vi "Part 2.vi"(11 "Input":string) -> (3 "Output":i64)   [LabVIEW 2021]
uses:
  <userlib>/_OpenG.lib/string/string.llb/Convert EOLs (String)__ogtk.vi
  Module/Module.lvclass
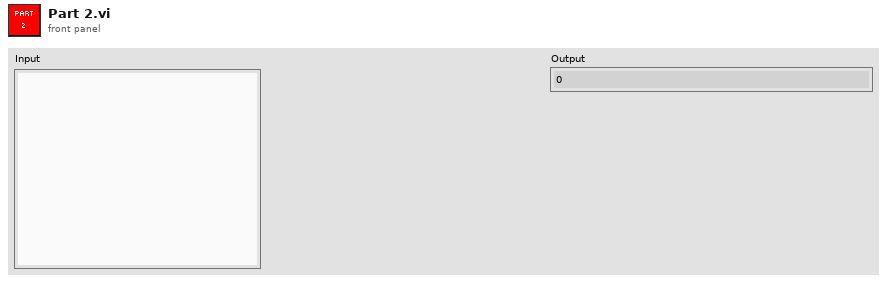
[diagram p1: front panel]
types:
  T1 = cluster{"From":string, "To":string, "Pulse":bool}
  T2 = cluster{"From":string, "To":string, "Pulse":bool}[]
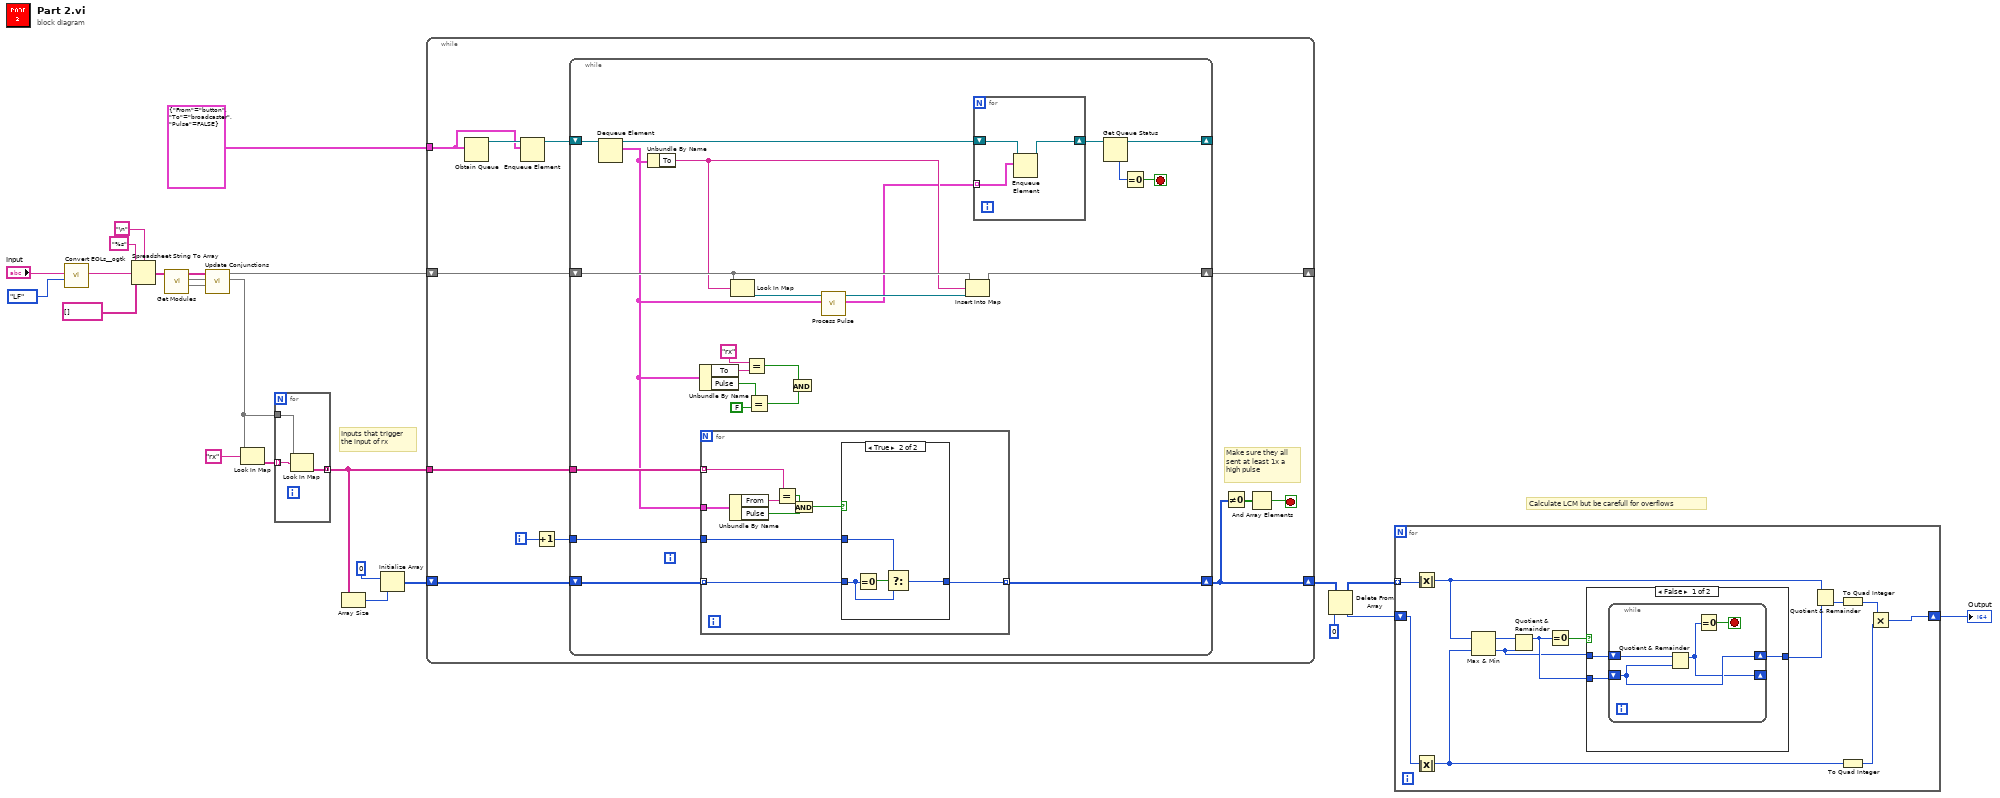
[diagram p0: block diagram]
diagram:
  # "Inputs that trigger\nthe input of rx"
  # "Calculate LCM but be carefull for overflows"
  n1 = call-poly <userlib>:"Convert EOLs__ogtk.vi"("Convert to:"=enum16{"CR", "LF", "CRLF"}."LF", "String in"="Input") -> ("String out"=w20:string)  [unwired: 9 in]
  n2 = Spreadsheet String To Array(delimiter (Tab)="\n", format string="%s", spreadsheet string=w20, array type (2D Dbl)=string[] []) -> (array=w18:string[])
  n3 = call "Get Modules.vi"("Module list in"=w18) -> ("Destination Map"=w15:map{string, string[]}, "Module Map"=w16:map{string, refnum<class "Module.lvclass">}, "Conjunctions out"=w17:string[])  [unwired: 8 in]
  n4 = call "Update Conjunctions.vi"("Destination Map in"=w15, "Module Map in"=w16, "Conjunctions in"=w17) -> ("Destination Map out"=w11:map{string, string[]}, "Module Map out"=w14:map{string, refnum<class "Module.lvclass">})  [unwired: 7 in]
  n5 = Look In Map(map=w11, key="rx") -> (value=w10:string[])  [unwired: 1 in, 1 out]
  n6 = for {
    tunnel: w11 -> [w25]
    tunnel: w10 -> [w27] mode=indexing
    tunnel: [w26] -> w9 mode=concatenating
    n7 = Look In Map(map=w25, key=w27) -> (value=w26:string[])  [unwired: 1 in, 1 out]
  }
  n8 = Array Size(array=w9) -> (size(s)=w8:i32)
  n9 = Initialize Array(i64 0, w8) -> (w6:i64[])
  n10 = while {
    shift-right: [w38] -> _
    shift-left: w14 -> [w39]
    tunnel: T1 {"From"="button", "To"="broadcaster", "Pulse"=FALSE} -> [w35]
    tunnel: w9 -> [w34]
    shift-right: [w32] -> w5
    shift-left: w6 -> [w33]
    i -> [w29]
    stop <- w30 stop-if-true
    # "Make sure they all\nsent at least 1x a\nhigh pulse"
    n11 = Obtain Queue(element data type=w35) -> (queue out=w37:refnum<queue>)  [unwired: 4 in, 2 out]
    n12 = Enqueue Element(queue=w37, element=w35) -> (queue out=w36:refnum<queue>)  [unwired: 2 in, 2 out]
    n13 = Increment(x=w29) -> (x+1=w28:i32)
    n14 = while {
      shift-right: [w55] -> w38
      shift-left: w39 -> [w58]
      shift-right: [w61] -> _
      shift-left: w36 -> [w60]
      tunnel: w34 -> [w44]
      shift-right: [w41] -> w32
      shift-left: w33 -> [w42]
      tunnel: w28 -> [w40]
      stop <- w51 stop-if-true
      n15 = Dequeue Element(queue=w60) -> (queue out=w54:refnum<queue>, element=w43:T1)  [unwired: 2 in, 2 out]
      n16 = Unbundle By Name(w43) -> ("To"=w57:string)
      n17 = Unbundle By Name(w43) -> ("To"=w50:string, "Pulse"=w48:bool)
      n18 = for {
        tunnel: w44 -> [w69] mode=indexing
        tunnel: w43 -> [w70]
        tunnel: w42 -> [w68] mode=indexing
        tunnel: [w67] -> w41 mode=indexing
        tunnel: w40 -> [w66]
        n19 = Unbundle By Name(w70) -> ("From"=w71:string, "Pulse"=w65:bool)
        n20 = Equal?(x=w69, y=w71) -> (x = y?=w64:bool)
        n21 = And(x=w64, y=w65) -> (x .and. y?=w63:bool)
        n22 = case shown="True" w63 {
          tunnel: w68 -> [w72 w73]
          tunnel: [w72 w74] -> w67
          tunnel: w66 -> [_ w75]
          frame False {
          }
          frame True {
            n23 = Equal To 0?(x=w73) -> (x = 0?=w76:bool)
            n24 = Select(t=w75, s=w76, f=w73) -> (s? t:f=w74:i64)
          }
        }
      }
      n25 = Look In Map(map=w58, key=w57) -> (value=w59:refnum<class "Module.lvclass">)  [unwired: 1 in, 1 out]
      n26 = Equal?(x="rx", y=w50) -> (x = y?=w45:bool)
      n27 = Equal?(x=w48, y=FALSE) -> (x = y?=w46:bool)
      n28 = And(x=w45, y=w46) -> ()  [unwired: 1 out]
      n29 = call-dynamic "Process Pulse.vi"("Input"=w43, "Module in"=w59) -> ("Outputs"=w52:T2, "Module out"=w56:refnum<class "Module.lvclass">)  [unwired: 7 in, 1 out]
      n30 = Insert Into Map(map in=w58, key=w57, value=w56) -> (map out=w55:map{string, refnum<class "Module.lvclass">})  [unwired: 2 out]
      n31 = for {
        shift-right: [w77] -> w53
        shift-left: w54 -> [w79]
        tunnel: w52 -> [w78] mode=indexing
        n32 = Enqueue Element(queue=w79, element=w78) -> (queue out=w77:refnum<queue>)  [unwired: 2 in, 2 out]
      }
      n33 = Get Queue Status(queue=w53) -> (queue out=w61:refnum<queue>, # elements in queue=w62:i32)  [unwired: 2 in, 6 out]
      n34 = Equal To 0?(x=w62) -> (x = 0?=w51:bool)
    }
    n35 = Not Equal To 0?(x=w32) -> (x != 0?=w31:bool[])
    n36 = And Array Elements(Boolean array=w31) -> (logical AND=w30:bool)
  }
  n37 = Delete From Array(array=w5, index=0) -> (deleted portion=w3:i64, array with subset deleted=w4:i64[])  [unwired: 1 in]
  n38 = for {
    tunnel: w4 -> [w89] mode=indexing
    shift-right: [w88] -> w1
    shift-left: w3 -> [w87]
    n39 = Absolute Value(x=w89) -> (abs(x)=w82:i64)
    n40 = Absolute Value(x=w87) -> (abs(x)=w81:i64)
    n41 = Max & Min(x=w82, y=w81) -> (max(x,y)=w83:i64, min(x,y)=w85:i64)
    n42 = Quotient & Remainder(x=w83, y=w85) -> (x-y*floor(x/y)=w86:i64)  [unwired: 1 out]
    n43 = Equal To 0?(x=w86) -> (x = 0?=w84:bool)
    n44 = case shown="False" w84 {
      tunnel: [w95 w100] -> w80
      tunnel: w85 -> [w94 w100]
      tunnel: w86 -> [w93 _]
      frame False {
        n45 = while {
          shift-right: [w97] -> w95
          shift-left: w94 -> [w98]
          shift-right: [w96] -> _
          shift-left: w93 -> [w97]
          stop <- w99 stop-if-true
          n46 = Quotient & Remainder(x=w98, y=w97) -> (x-y*floor(x/y)=w96:i64)  [unwired: 1 out]
          n47 = Equal To 0?(x=w96) -> (x = 0?=w99:bool)
        }
      }
      frame True {
      }
    }
    n48 = Quotient & Remainder(x=w82, y=w80) -> (floor(x/y)=w92:i64)  [unwired: 1 out]
    n49 = To Quad Integer(1:w92) -> (0:w90:i64)
    n50 = To Quad Integer(1:w81) -> (0:w91:i64)
    n51 = Multiply(x=w90, y=w91) -> (x*y=w88:i64)
  }
  "Output" <- w1
